vi "Get Stack Voltage.vi"(8 "error in":errorcluster, 10 "MCU Selector":T1, 11 "HSU MCU V2 Monitor CFG in":refnum<class "HSU MCU V2 Monitor CFG.lvclass">) -> (0 "error out":errorcluster, 2 "Voltage DC":dbl format="%#_g V", 3 "HSU MCU V2 Monitor CFG out":refnum<class "HSU MCU V2 Monitor CFG.lvclass">)   [LabVIEW 2023, in "HSU MCU V2 Monitor CFG.lvclass"]
uses:
  HSU MCU V2 Monitor CFG.lvclass
  HSU MCU V2 Monitor CFG.lvclass/HSU MCU V2 Monitor CFG.ctl
  Protocols/ICAN/ICAN.lvclass
  MCU Selector.ctl
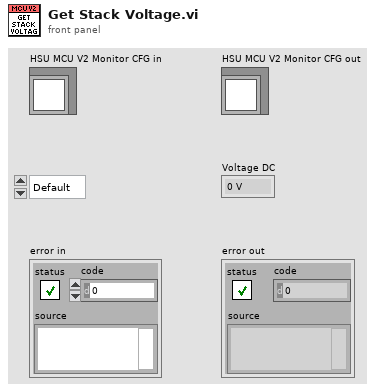
[diagram p1: front panel]
types:
  T1 = typedef "MCU Selector.ctl" = enum16{"Default", "MCU1", "MCU2", "MCU3", "MCU4", "MCU5", "MCU6", "MCU7", "MCU8"}
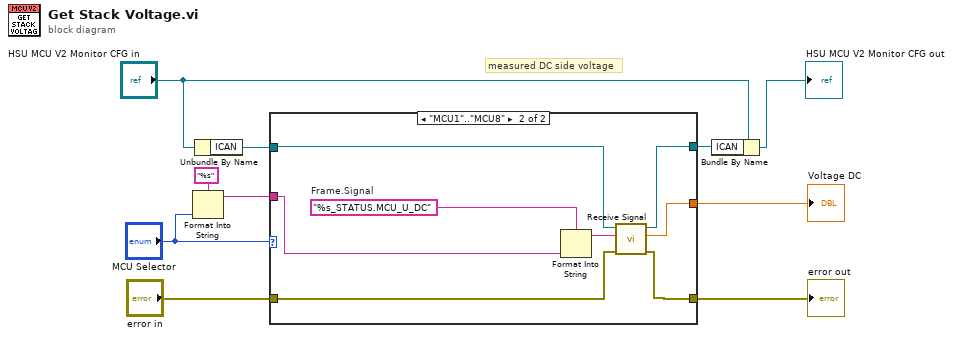
[diagram p0: block diagram]
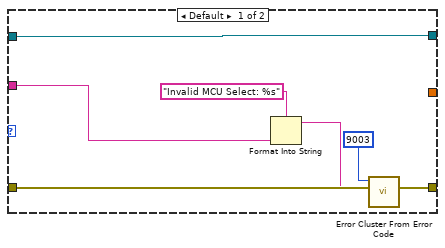
[diagram p2: hidden frame]
diagram:
  # "measured DC side voltage"
  n1 = Format Into String(format string="%s", "MCU Selector") -> (resulting string=w8:string)  [unwired: 2 in, 1 out]
  n2 = Unbundle By Name("HSU MCU V2 Monitor CFG in") -> ("ICAN"=w7:refnum<class "ICAN.lvclass">)
  n3 = case shown="\"MCU1\"..\"MCU8\"" "MCU Selector" {
    tunnel: "error in" -> [w17 w23]
    tunnel: [w16 w22] -> w5
    tunnel: w8 -> [w12 w25]
    tunnel: w7 -> [w11 w24]
    tunnel: [w11 w21] -> w4
    tunnel: [_ w18] -> w1
    frame Default {
      n4 = Format Into String(format string="Invalid MCU Select: %s" ("error message (\"\")"), w12) -> (resulting string=w14:string)  [unwired: 2 in, 1 out]
      n5 = call <vilib>:"Error Cluster From Error Code.vi"("error in (no error)"=w17, "error message (\"\")"=w14, "error code (0)"=9003) -> ("error out"=w16:errorcluster)  [unwired: 6 in]
    }
    frame "MCU1".."MCU8" {
      w20 = "%s_STATUS.MCU_U_DC"  # Frame.Signal
      n6 = Format Into String(format string=w20, w25) -> (resulting string=w19:string)  [unwired: 2 in, 1 out]
      n7 = call-dynamic "Receive Signal.vi"("error in"=w23, "Frame.Signal"=w19, "ICommunicate in"=w24) -> ("error out"=w22:errorcluster, "Value"=w18:dbl, "ICommunicate out"=w21:refnum<class "ICAN.lvclass">)  [unwired: 6 in]
    }
  }
  "error out" <- w5
  "Voltage DC" <- w1
  n8 = Bundle By Name(cluster="HSU MCU V2 Monitor CFG in", "ICAN"=w4) -> (→"HSU MCU V2 Monitor CFG out":refnum<class "HSU MCU V2 Monitor CFG.lvclass">)
